vi "SDI Send Cmd.vi"(6 "CheckCRC":u8, 7 "pCommand":string, 8 "error in (no error)":errorcluster, 9 "SDIIndex":u8, 10 "DevIndex":i32, 11 "DevType":i32) -> (0 "error out":errorcluster, 2 "function return":i32, 3 "pRespond":string)   [LabVIEW 2012, in "ControlSDI.lvlib"]
doc: "int WINAPI SDI_SendCmd(int DevType, int DevIndex, unsigned char SDIIndex,unsigned char *pCommand,unsigned char *pRespond,unsigned char CheckCRC);"
uses:
  ControlSDI.lvlib
  Ginkgo_Driver.dll
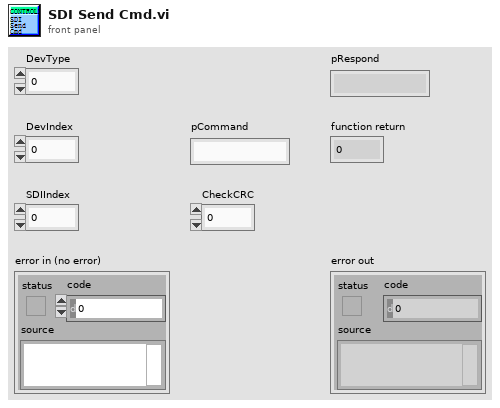
[diagram p1: front panel]
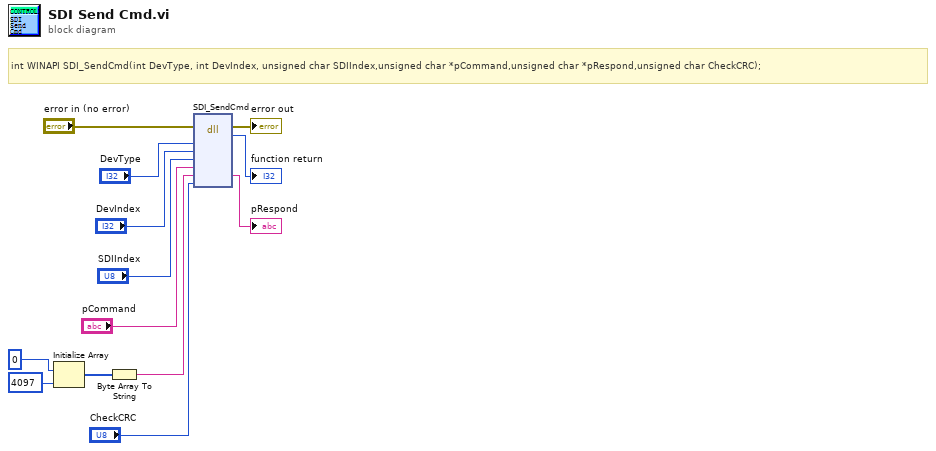
[diagram p0: block diagram]
diagram:
  # "int WINAPI SDI_SendCmd(int DevType, int DevIndex, unsigned char SDIIndex,unsigned char *pCommand,unsigned char *pRespond,unsigned char CheckCRC);"
  n1 = Initialize Array(u8 0 ("element"), 4097 ("dimension size")) -> (w8:u8[])
  n2 = Byte Array To String(unsigned byte array=w8) -> (string=w7:string)
  n3 = dll-call lib="E:/Project/vt_ginkgo/truck/Ginkgo Driver/vs2010/Ginkgo_USB-I2C_API_v2.0.3.0/lib/labview_64bit/ControlSDI/Ginkgo_Driver.*" fn="SDI_SendCmd"(error in="error in (no error)", "DevType"="DevType", "DevIndex"="DevIndex", "SDIIndex"="SDIIndex", "pCommand"="pCommand", "pRespond"=w7, "CheckCRC"="CheckCRC") -> (error out=→"error out":errorcluster, →"function return":i32, "pRespond"=→"pRespond":string)  [unwired: 7 in, 1 out]
